vi "Clear Buffer.vi"   [LabVIEW 2011, in "CAN FD.lvlib"]
uses:
  CAN FD.lvlib
  Typedef/CAN Data.ctl
types:
  T1 = typedef "CAN FD.lvlib/CAN Data.ctl" = cluster{"SystemTime":timestamp, "HwTime":dbl, "Channel":u8, "ID":u32, "CANType":i16, "Direction":i16, "Remote":bool, "Ext":bool, "Len":u8, "Data":u8[], "Success":bool}
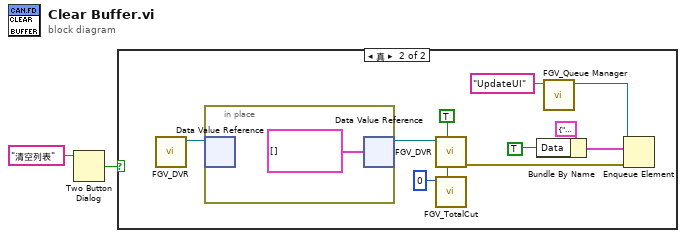
[diagram p0: block diagram]
diagram:
  n1 = Two Button Dialog(message="清空列表" ("消息")) -> (T button?=w1:bool)  [unwired: 2 in]
  n2 = case shown="真" w1 {
    frame False {
    }
    frame True {
      w3 = TRUE ("Set")
      n3 = call "FGV_DVR.vi"() -> ("DVR"=w12:refnum<data-value>)  [unwired: 10 in, 1 out]
      n4 = in-place {
        n5 = in-place-dvr #1(w12) -> ()  [unwired: 2 out]
        n6 = in-place-dvr #1(T1[] [] ("数据值")) -> (w11:refnum<data-value>)  [unwired: 1 out]
      }
      n7 = call "FGV_DVR.vi"("Set"=w3, "DVR"=w11) -> ("error out"=w5:errorcluster)  [unwired: 8 in, 1 out]
      n8 = call "FGV_TotalCut.vi"("Set"=w3, "Total cut"=0 ("TotalCount")) -> ()  [unwired: 8 in, 2 out]
      n9 = Bundle By Name(cluster=cluster{"ID":string, "Data":variant} {"ID"="Update", "Data"=variant} ("元素"), "Data"=TRUE) -> (w8:cluster{"ID":string, "Data":variant})
      n10 = call "FGV_Queue Manager.vi"("Name"="UpdateUI") -> ("Queue"=w6:refnum<queue>)  [unwired: 8 in, 2 out]
      n11 = Enqueue Element(queue=w6, element=w8, error in (no error)=w5) -> ()  [unwired: 1 in, 3 out]
    }
  }
